vi "MPS_HV_PowerSupplyInterface.vi"() -> ()   [LabVIEW 2013]
uses:
  <vilib>/Instr/_visa.llb/VISA Configure Serial Port (Instr).vi
panel:
  out "Reported currents":T1
  out "Reported voltages":T1
  in  "Voltage Slew Rate (V/s)":dbl
  out "error out":errorcluster
  in  "Resend all":bool
  in  "VISA resource name":refnum<visa-resource-name>="COM11"
  in  "Stop and zero supplies":bool
  out "x != y?":T2
  in  "Power supply \ncontrol voltages":T1 {"Supply 5" min=0.0 max=5000.0 step=0.1 scale=0.0..5000.0 scale format="%#_4p"; "Supply 4" min=0.0 max=5000.0 step=0.1 scale=0.0..5000.0 scale format="%#_4p"; "Supply 3" min=0.0 max=5000.0 step=0.1 scale=0.0..5000.0 scale format="%#_4p"; "Supply 2" min=0.0 max=5000.0 step=0.1 scale=0.0..5000.0 scale format="%#_4p"; "Supply 1" min=0.0 max=5000.0 step=0.1 scale=0.0..5000.0 scale format="%#_4p"}
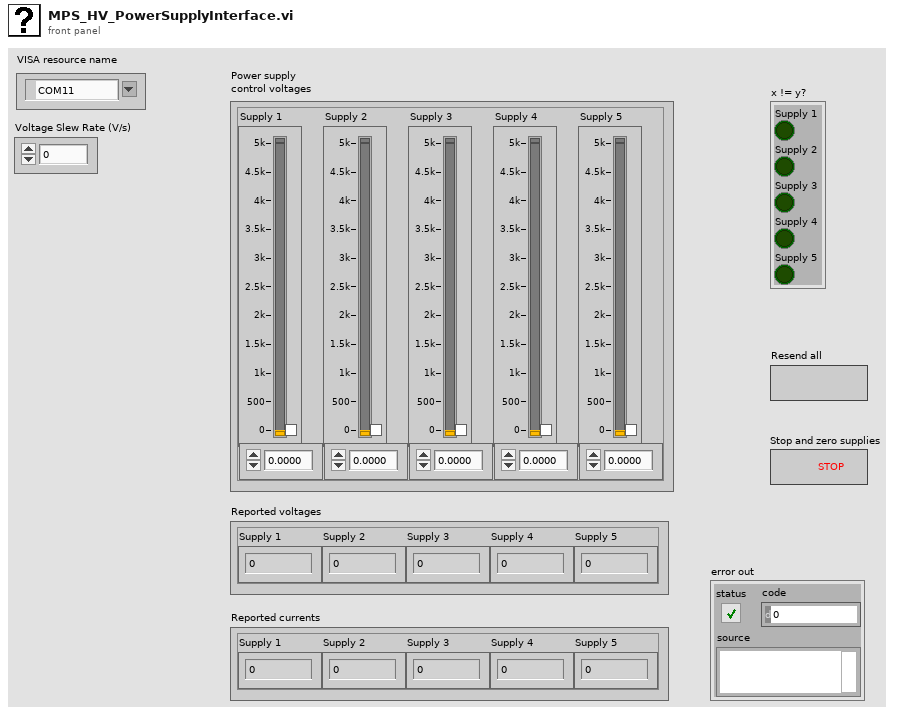
[diagram p1: front panel]
types:
  T1 = cluster{"Supply 1":dbl, "Supply 2":dbl, "Supply 3":dbl, "Supply 4":dbl, "Supply 5":dbl}
  T2 = cluster{"Supply 1":bool, "Supply 2":bool, "Supply 3":bool, "Supply 4":bool, "Supply 5":bool}
  T3 = cluster{"baud rate":u32, "data bits":u16, "parity":enum16{"None", "Odd", "Even", "Mark", "Space"}, "stop bits":u16, "flow control":u16}
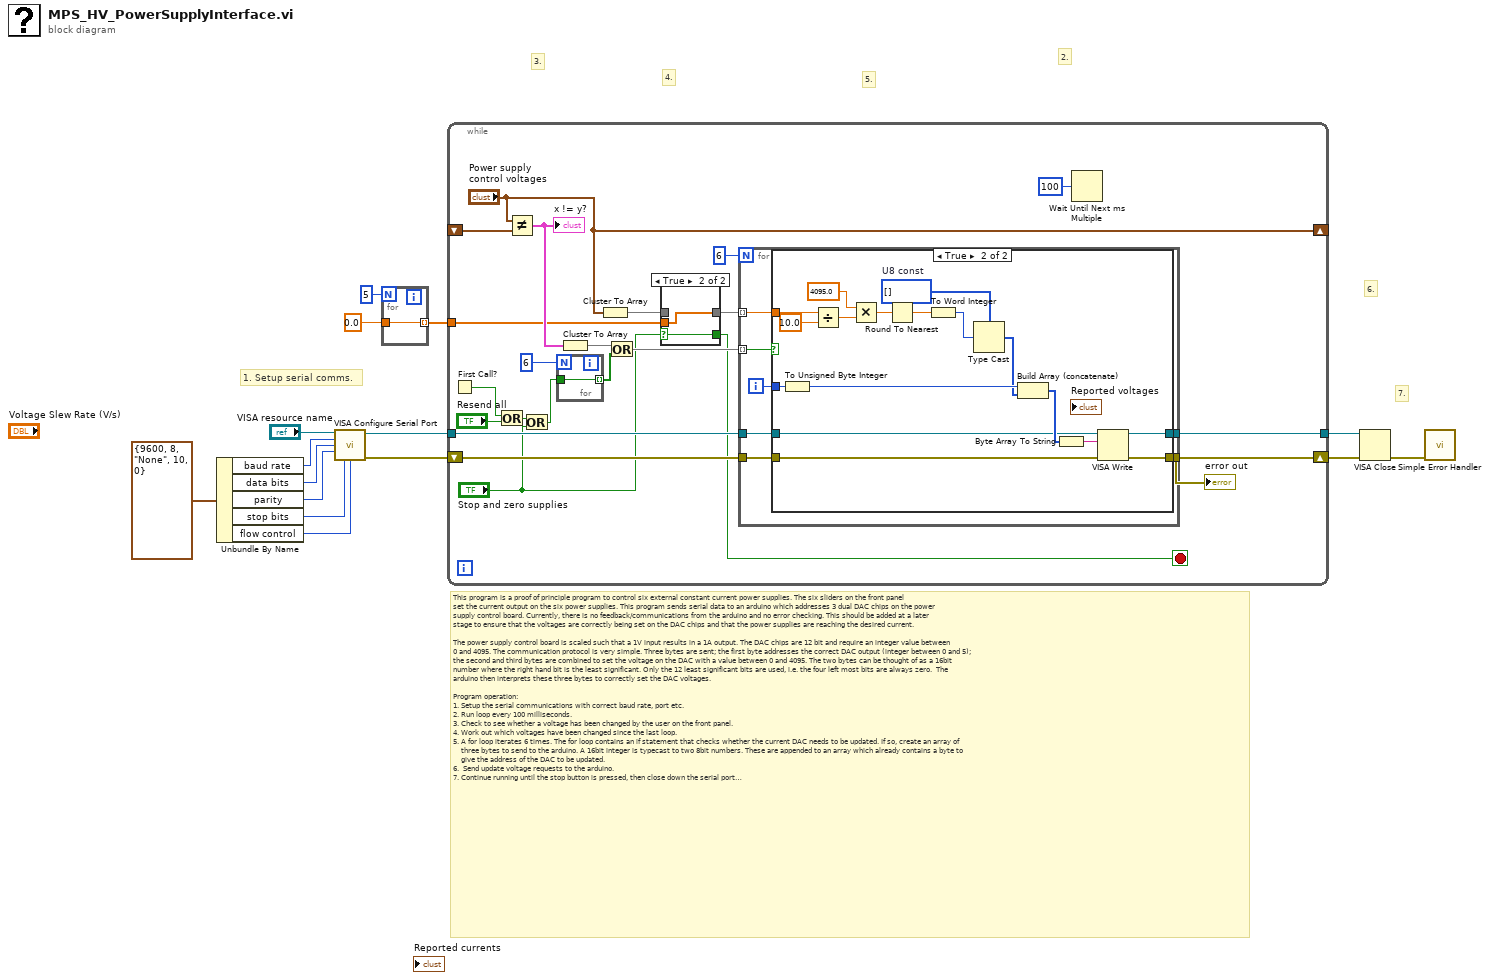
[diagram p0: block diagram]
diagram:
  # "7."
  # "6."
  # "5."
  # "4."
  # "2."
  # "3."
  # "This program is a proof of principle program to control six external constant current power supplies. The six sliders on the front panel\nset the current output on the six power supplies. This program sends serial data to an arduino which addresses 3 dual DAC chips on the power\nsupply control board. Currently, there is no feedback/communications from the arduino and no error checking. This should be added at a later \nstage to ensure that the voltages are correctly being set on the DAC chips and that the power supplies are reaching the desired current.\n\nThe power supply control board is scaled such that a 1V input results in a 1A output. The DAC chips are 12 bit and require an integer value between\n0 and 4095. The communication protocol is very simple. Three bytes are sent; the first byte addresses the correct DAC output (integer between 0 and 5);\nthe second and third bytes are combined to set the voltage on the DAC with a value between 0 and 4095. The two bytes can be thought of as a 16bit \nnumber where the right hand bit is the least significant. Only the 12 least significant bits are used, i.e. the four left most bits are always zero.  The \narduino then interprets these three bytes to correctly set the DAC voltages.\n\nProgram operation:\n1. Setup the serial communications with correct baud rate, port etc.\n2. Run loop every 100 milliseconds.\n3. Check to see whether a voltage has been changed by the user on the front panel.\n4. Work out which voltages have been changed since the last loop.\n5. A for loop iterates 6 times. The for loop contains an if statement that checks whether the current DAC needs to be updated. If so, create an array of \n    three bytes to send to the arduino. A 16bit integer is typecast to two 8bit numbers. These are appended to an array which already contains a byte to \n    give the address of the DAC to be updated.\n6.  Send update voltage requests to the arduino.\n7. Continue running until the stop button is pressed, then close down the serial port.\n\nWhen the program is run for the first time, the first call? function next to the Resend all control ensures that all six channels are reinitialised to 0."
  # "1. Setup serial comms."
  n1 = Unbundle By Name(T3 {"baud rate"=9600, "data bits"=8, "parity"=enum."None", "stop bits"=10, "flow control"=0} ("Serial Settings")) -> ("baud rate"=w12:u32, "data bits"=w11:u16, "parity"=w10:enum16{"None", "Odd", "Even", "Mark", "Space"}, "stop bits"=w9:u16, "flow control"=w8:u16)
  n2 = call-poly "VISA Configure Serial Port"("VISA resource name"="VISA resource name", "baud rate (9600)"=w12, "data bits (8)"=w11, "parity (0:none)"=w10, "stop bits (10: 1 bit)"=w9, "flow control (0:none)"=w8) -> ("VISA resource name out"=w4:refnum<visa-resource-name>, "error out"=w5:errorcluster)  [unwired: 3 in, 5 out]
  n3 = for {
    N: 5 -> [_]
    tunnel: 0.0 ("y") -> [w16]
    tunnel: [w16] -> w1 mode=indexing
  }
  n4 = while {
    shift-right: ["Power supply \ncontrol voltages"] -> _
    shift-left: _ -> [w38]
    tunnel: w4 -> [w29]
    tunnel: [w26] -> w6
    tunnel: w1 -> [w21]
    shift-right: [w27] -> w7
    shift-left: w5 -> [w28]
    stop <- w20 stop-if-true
    n5 = First Call?() -> (First Call?: T/F=w24:bool)
    n6 = Or(x=w24, y="Resend all") -> (x .or. y?=w19:bool)
    n7 = Not Equal?(x="Power supply \ncontrol voltages", y=w38) -> (x != y?=w36:T2)
    "x != y?" <- w36
    n8 = Or(x=w19, y="Stop and zero supplies") -> (x .or. y?=w17:bool)
    n9 = for {
      N: 6 -> [_]
      tunnel: w17 -> [w43]
      tunnel: [w43] -> w31 mode=indexing
    }
    n10 = Cluster To Array(cluster=w36) -> (array=w34:bool[])
    n11 = Cluster To Array(cluster="Power supply \ncontrol voltages") -> (array=w23:dbl[])
    n12 = Or(x=w34, y=w31) -> (x .or. y?=w33:bool[])
    n13 = case shown="True" "Stop and zero supplies" {
      selector: "Stop and zero supplies" -> [w39 w41]
      tunnel: w23 -> [w40 _]
      tunnel: [w40 w42] -> w22
      tunnel: w21 -> [_ w42]
      tunnel: [w39 w41] -> w20
      frame False {
      }
      frame True {
      }
    }
    n14 = for {
      N: 6 -> [_]
      tunnel: w33 -> [w50] mode=indexing
      tunnel: w22 -> [w49] mode=indexing
      tunnel: w29 -> [w47]
      tunnel: w28 -> [w46]
      tunnel: [w45] -> w27
      tunnel: [w44] -> w26
      i -> [w48]
      n15 = case shown="True" w50 {
        tunnel: w49 -> [_ w68]
        tunnel: w48 -> [_ w69]
        tunnel: w47 -> [w52 w55]
        tunnel: w46 -> [w51 w56]
        tunnel: [w51 w54] -> w45
        tunnel: [w52 w53] -> w44
        frame False {
        }
        frame True {
          w59 = u8[] []  # U8 const
          n16 = To Unsigned Byte Integer(number=w69) -> (unsigned 8bit integer=w63:u8)
          n17 = Divide(x=w68, y=10.0) -> (x/y=w66:dbl)
          n18 = Multiply(x=4095.0 ("y"), y=w66) -> (x*y=w64:dbl)
          n19 = Round To Nearest(number=w64) -> (nearest integer value=w62:dbl)
          n20 = To Word Integer(number=w62) -> (16bit integer=w61:i16)
          n21 = Type Cast(type=w59, x=w61) -> (*(type *) &x=w60:u8[])
          n22 = Build Array (concatenate)(w63, w60) -> (w58:u8[])
          n23 = Byte Array To String(unsigned byte array=w58) -> (string=w57:string)
          n24 = VISA Write(VISA resource name=w55, write buffer=w57, error in (no error)=w56) -> (VISA resource name out=w53:refnum<visa-resource-name>, error out=w54:errorcluster)  [unwired: 1 out]
        }
      }
    }
    "error out" <- w27
    n25 = Wait Until Next ms Multiple(millisecond multiple=u32 100) -> ()  [unwired: 1 out]
  }
  n26 = VISA Close(VISA resource name=w6, error in (no error)=w7) -> (error out=w14:errorcluster)
  n27 = call <vilib>:"Simple Error Handler.vi"("error in (no error)"=w14) -> ()  [unwired: 1 in, 8 out]
